vi "Playback Latency Compare Example.vi"() -> ()   [LabVIEW 2020]
doc: "Simple example of audio device playback of a file decoded with G-Audio."
uses:
  Controls/Audio Device Config.ctl
  Controls/Audio Device Format.ctl
  Controls/Audio Device Info.ctl
  Controls/Audio Device Type.ctl
  <vilib>/sound2/lvsound2.llb/Sampling Mode.ctl
  <vilib>/sound2/lvsound2.llb/Sound Data Format.ctl
  a109801a-35bf-4c7b-a749-e9ca6f5be5a9.vi
  31459d8e-8b05-43dc-a9de-d0cb0458a0b2.vi
  7384a574-0dee-437e-8049-4055a9225864.vi
  9545a255-db38-479b-bcdc-619f4ee8d9ed.vi
  Private/Result To Error.vi
  a109801a-35bf-4c7b-a749-e9ca6f5be5a9.vi/56465d8a-8d83-4810-9820-5ab2fa709974.vi
  31459d8e-8b05-43dc-a9de-d0cb0458a0b2.vi/15efb94c-0eeb-49fd-9ff3-8ea0cffaf39a.vi
  9545a255-db38-479b-bcdc-619f4ee8d9ed.vi/4dfb5711-8d81-45a3-b3db-a84d40650863.vi
  9545a255-db38-479b-bcdc-619f4ee8d9ed.vi/c8869513-30c6-44f2-a2d3-73232fe63870.vi
  9545a255-db38-479b-bcdc-619f4ee8d9ed.vi/4dfb5711-8d81-45a3-b3db-a84d40650863.vi/4b7b629c-2e91-4160-9820-a26af8f6e677.vi
  9545a255-db38-479b-bcdc-619f4ee8d9ed.vi/c8869513-30c6-44f2-a2d3-73232fe63870.vi/4b7b629c-2e91-4160-9820-a26af8f6e677.vi
  <vilib>/Utility/error.llb/Error Cluster From Error Code.vi
  Private/Copy Data.vi
  <vilib>/sound2/lvsound2.llb/Sound Output Write (I16).vi
  <vilib>/Utility/Data Type/Get Numeric Information.vi
  G-Audio.lvlib
panel:
  out "error out 3":errorcluster
  out "Now Playing:":string
  out "Duration":string
  out "Sample Length":u64
  out "Audio Info":T1
  out "error out":errorcluster
  in  "Stop":bool
  # "This example demonstrates the reduced latency of G-Audio (WASAPI) as compared to LabVIEW Sound (DirectSound).\nIt's not a perfect comparison, and other factors can introduce latency between the two playback methods. In general\nthough the WASAPI backend exhibits lower latency than DirectSound.\n\nInstructions:\n1. Run the VI.\n2. Select an audio file to play (music with sharp attacks will be most noticable).\n3. The file will begin playback using both G-Audio and LabVIEW Sound.\n    G-Audio will be played on the left channel, and LabVIEW Sound on the right.\n4. Listen with headphones for a slight phase shift between the left and right channels.\n5. Record the audio in Audacity using the loopback adapter, and observe the phase difference."
  # "G"
  # "-Audio"
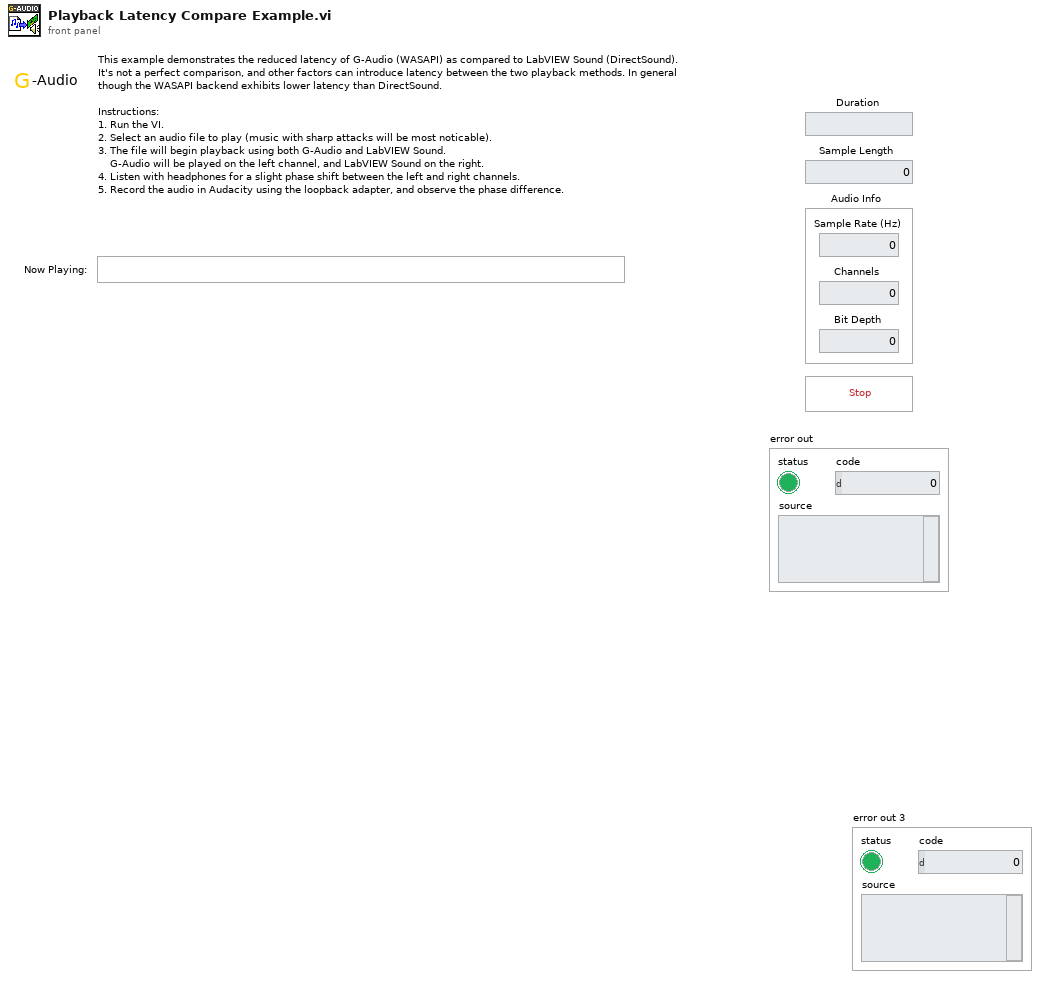
[diagram p1: front panel]
types:
  T1 = cluster{"Sample Rate (Hz)":u32, "Channels":u32, "Bit Depth":u32}
  T2 = typedef "Sound Data Format.ctl" = cluster{"sample rate (S/s)":dbl, "number of channels":i32, "bits per sample":i32}
  T3 = typedef "Sampling Mode.ctl" = i32
  T4 = typedef "G-Audio.lvlib/Audio Device Info.ctl" = cluster{"Name":string, "ID":u8[], "Device Type":T5}
  T5 = typedef "G-Audio.lvlib/Audio Device Type.ctl" = enum16{"(None)", "Playback", "Capture", "Duplex", "Loopback"}
  T6 = typedef "G-Audio.lvlib/Audio Device Config.ctl" = cluster{"Sample Rate (Hz)":u32, "Channels":u32, "Format":T7, "Exclusive Mode":bool}
  T7 = typedef "G-Audio.lvlib/Audio Device Format.ctl" = enum16{"Native", "U8", "I16", "I32", "SGL"}
  T8 = typedef "G-Audio.lvlib/Audio File Info.ctl" = cluster{"Sample Rate (Hz)":u32, "Channels":u32, "Bit Depth":u32}
  T9 = typedef "G-Audio.lvlib/Audio Device Refnum.ctl" = refnum<file>
  T10 = typedef "Sound Output Task ID.ctl" = u32
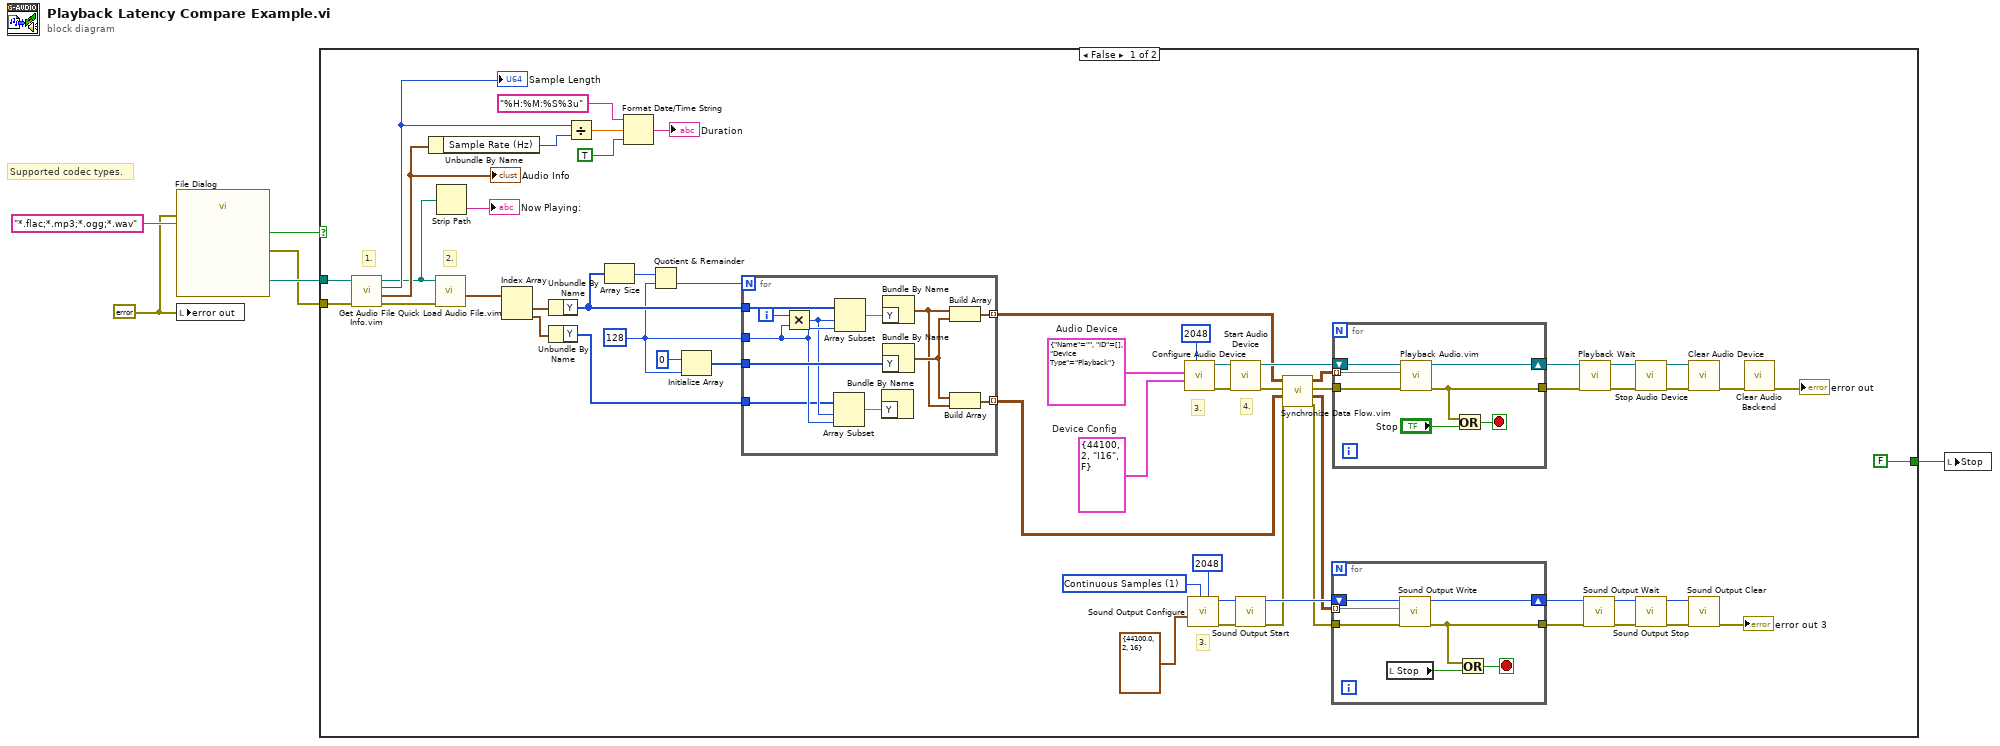
[diagram p0: block diagram]
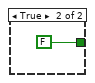
[diagram p2: hidden frame]
diagram:
  w2 = errorcluster {"status"=FALSE, "code"=0, "source"=""} ("error out")
  # "Supported codec types."
  n1 = call "File Dialog"("error in"=w2, "pattern (all files)"="*.flac;*.mp3;*.ogg;*.wav") -> ("selected path"=w5:path, "cancelled"=w4:bool, "error out"=w3:errorcluster)  [unwired: 10 in, 1 out]
  n2 = local write "error out"(w2) -> ()
  n3 = case shown="False" w4 {
    tunnel: w5 -> [w58 _]
    tunnel: w3 -> [w64 _]
    tunnel: [FALSE ("Stop") FALSE ("Stop")] -> w1
    frame False {
      w18 = 128 ("y")
      w39 = T3 1 items=["Finite Samples", "Continuous Samples"] ("sample mode")
      w41 = T4 {"Name"="", "ID"=[], "Device Type"=enum."Playback"}  # Audio Device
      w42 = T6 {"Sample Rate (Hz)"=44100, "Channels"=2, "Format"=enum."I16", "Exclusive Mode"=FALSE}  # Device Config
      # "3."
      # "4."
      # "3."
      # "2."
      # "1."
      n4 = call "Get Audio File Info.vim"("error in (no error)"=w64, "Path In"=w58) -> ("error out"=w63:errorcluster, "Audio File Info"=w55:T8, "PCM Frame Length"=w56:u64, "Path Out"=w50:path)  [unwired: 5 in, 1 out]
      "Audio Info" <- w55
      "Sample Length" <- w56
      n5 = Unbundle By Name(w55) -> ("Sample Rate (Hz)"=w54:u32)
      n6 = call "Quick Load Audio File.vim"("error in (no error)"=w63, "Path"=w50) -> ("data"=w22:waveform(i16)[])  [unwired: 4 in, 5 out]
      n7 = Strip Path(path=w50) -> (name=→"Now Playing:":string)  [unwired: 1 out]
      n8 = Index Array(array=w22) -> (element #1=w21:waveform(i16), element #2=w15:waveform(i16))  [unwired: 2 in]
      n9 = Unbundle By Name(w21) -> ("Y"=w19:i16[])
      n10 = Unbundle By Name(w15) -> ("Y"=w14:i16[])
      n11 = Divide(x=w56, y=w54) -> (x/y=w53:dbl)
      n12 = Array Size(array=w19) -> (size(s)=w23:i32)
      n13 = Format Date/Time String(time format string (%c)="%H:%M:%S%3u", seconds (now)=w53, UTC format=TRUE) -> (date/time string=→"Duration":string)
      n14 = Quotient & Remainder(x=w23, y=w18) -> (floor(x/y)=w20:i32)  [unwired: 1 out]
      n15 = Initialize Array(i16 0 ("y"), w18) -> (w16:i16[])
      n16 = for {
        N: w20 -> [_]
        tunnel: w19 -> [w76]
        tunnel: w18 -> [w70]
        tunnel: w16 -> [w73]
        tunnel: [w72] -> w11 mode=indexing
        tunnel: w14 -> [w68]
        tunnel: [w67] -> w9 mode=indexing
        i -> [w74]
        n17 = Multiply(x=w74, y=w70) -> (x*y=w69:i32)
        n18 = Array Subset(array=w68, index=w69, length=w70) -> (w71:i16[])
        n19 = Array Subset(array=w76, index=w69, length=w70) -> (w75:i16[])
        n20 = Bundle By Name("Y"=w71) -> ()  [unwired: 1 in, 1 out]
        n21 = Bundle By Name("Y"=w75) -> (w65:waveform(i16))  [unwired: 1 in]
        n22 = Bundle By Name("Y"=w73) -> (w66:waveform(i16))  [unwired: 1 in]
        n23 = Build Array(w65, w66) -> (w72:waveform(i16)[])
        n24 = Build Array(w66, w65) -> (w67:waveform(i16)[])
      }
      n25 = call "Configure Audio Device.vi"("Buffer Size (4096)"=2048 ("number of samples/ch"), "Device Config"=w42, "Audio Device"=w41) -> ("error out"=w48:errorcluster, "Audio Device Refnum"=w47:T9)  [unwired: 7 in]
      n26 = call <vilib>:"Sound Output Configure.vi"("number of samples/ch"=2048, "sample mode"=w39, "sound format"=T2 {"sample rate (S/s)"=44100.0, "number of channels"=2, "bits per sample"=16}) -> ("error out"=w31:errorcluster, "task ID"=w36:T10)  [unwired: 7 in]
      n27 = call "Start Audio Device.vi"("error in (no error)"=w48, "Audio Device Refnum In"=w47) -> ("error out"=w13:errorcluster, "Audio Device Refnum Out"=w60:T9)  [unwired: 8 in]
      n28 = call <vilib>:"Sound Output Start.vi"("error in (no error)"=w31, "task ID"=w36) -> ("error out"=w30:errorcluster, "task ID out"=w32:T10)  [unwired: 8 in]
      n29 = call "Synchronize Data Flow.vim"("input 4"=w30, "input 3"=w9, "input 2"=w13, "input 1"=w11) -> ("output 4"=w29:errorcluster, "output 3"=w8:waveform(i16)[][], "output 2"=w12:errorcluster, "output 1"=w10:waveform(i16)[][])
      n30 = for {
        shift-right: [w82] -> w38
        shift-left: w32 -> [w83]
        tunnel: w29 -> [w79]
        tunnel: [w81] -> w27
        tunnel: w8 -> [w77] mode=indexing
        stop <- w78 stop-if-true
        n31 = local read "Stop"() -> (w80:bool)
        n32 = call-poly <vilib>:"Sound Output Write.vi"("error in (no error)"=w79, "data"=w77, "task ID"=w83) -> ("error out"=w81:errorcluster, "task ID out"=w82:T10)  [unwired: 7 in]
        n33 = Or(x=w81, y=w80) -> (x .or. y?=w78:bool)
      }
      n34 = for {
        shift-right: [w89] -> w44
        shift-left: w60 -> [w90]
        tunnel: w12 -> [w86]
        tunnel: [w87] -> w28
        tunnel: w10 -> [w84] mode=indexing
        stop <- w85 stop-if-true
        n35 = call "Playback Audio.vim"("error in (no error)"=w86, "Audio Data"=w84, "Audio Device Refnum In"=w90) -> ("error out"=w87:errorcluster, "Audio Device Refnum Out"=w89:T9)  [unwired: 7 in]
        n36 = Or(x=w87, y="Stop") -> (x .or. y?=w85:bool)
      }
      n37 = call "Playback Wait.vi"("error in (no error)"=w28, "Audio Device Refnum In"=w44) -> ("error out"=w45:errorcluster, "Audio Device Refnum Out"=w43:T9)  [unwired: 8 in]
      n38 = call <vilib>:"Sound Output Wait.vi"("error in (no error)"=w27, "task ID"=w38) -> ("error out"=w25:errorcluster, "task ID out"=w37:T10)  [unwired: 8 in]
      n39 = call "Stop Audio Device.vi"("error in (no error)"=w45, "Audio Device Refnum In"=w43) -> ("error out"=w61:errorcluster, "Audio Device Refnum Out"=w62:T9)  [unwired: 8 in]
      n40 = call <vilib>:"Sound Output Stop.vi"("error in (no error)"=w25, "task ID"=w37) -> ("error out"=w24:errorcluster, "task ID out"=w26:T10)  [unwired: 8 in]
      n41 = call "Clear Audio Device.vi"("error in (no error)"=w61, "Audio Device Refnum In"=w62) -> ("error out"=w59:errorcluster)  [unwired: 9 in]
      n42 = call <vilib>:"Sound Output Clear.vi"("error in (no error)"=w24, "task ID"=w26) -> ("error out"=→"error out 3":errorcluster)  [unwired: 9 in]
      n43 = call "Clear Audio Backend.vi"("error in (no error)"=w59) -> ("error out"=→"error out":errorcluster)  [unwired: 10 in]
    }
    frame True {
    }
  }
  n44 = local write "Stop"(w1) -> ()
